vi "Sign with Certificate.vi"(6 "url":string, 7 "tsa":string, 8 "error in (no error)":errorcluster, 9 "store":string, 10 "certname":string, 11 "filepath":string) -> (0 "error out":errorcluster)   [LabVIEW 2020, in "CodeSignAPI.lvlib"]
doc: "ni_sign_w_cert(const char *filepath, const char *certname, const char *store,\n const char *tsa, const char *url);"
uses:
  <vilib>/AppBuilder/CodeSignAPI/CodeSignAPI.lvlib
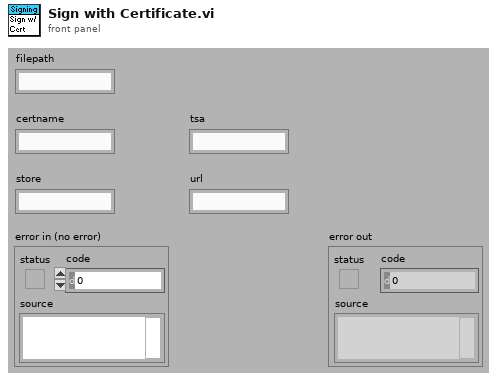
[diagram p1: front panel]
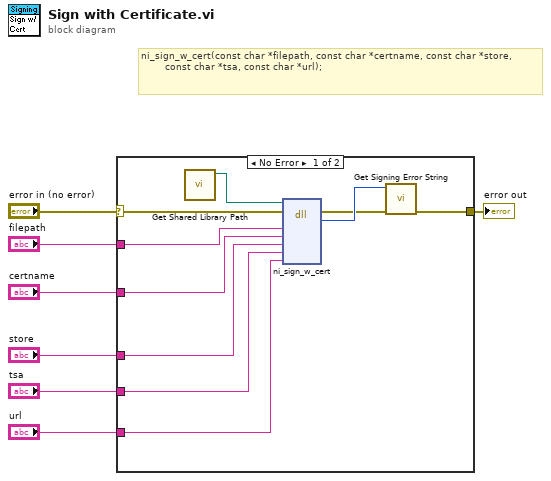
[diagram p0: block diagram]
diagram:
  # "ni_sign_w_cert(const char *filepath, const char *certname, const char *store,\n\t\t\t\t\t\t\t const char *tsa, const char *url);"
  n1 = case shown="No Error" "error in (no error)" {
    selector: "error in (no error)" -> [w12 w18]
    tunnel: "filepath" -> [w17 _]
    tunnel: "certname" -> [w16 _]
    tunnel: "store" -> [w15 _]
    tunnel: "url" -> [w14 _]
    tunnel: "tsa" -> [w13 _]
    tunnel: [w8 w18] -> w2
    frame No Error {
      n2 = call <vilib>:"Get Shared Library Path.vi"() -> ("shared library path"=w11:path)  [unwired: 1 in, 10 out]
      n3 = dll-call lib="?" fn="ni_sign_w_cert"(path in=w11, error in=w12, "filepath"=w17, "certname"=w16, "store"=w15, "tsa"=w13, "url"=w14) -> (error out=w9:errorcluster, "return type"=w10:i64)  [unwired: 6 in, 1 out]
      n4 = call <vilib>:"Get Signing Error String.vi"("error in (no error)"=w9, "NICSGN_ERROR"=w10) -> ("error out"=w8:errorcluster)  [unwired: 9 out]
    }
    frame Error {
    }
  }
  "error out" <- w2
